vi "Sauna_9642_FPGA_Main.vi"() -> ()   [LabVIEW 2019]
uses:
  <vilib>/LabVIEW Targets/FPGA/cRIO/shared/nicrio_ModuleControls/nicrio_cRIO-9219_ConversionTime.ctl
  <vilib>/LabVIEW Targets/FPGA/cRIO/shared/nicrio_ModuleControls/nicrio_cRIO-9219_FullBridgeRange.ctl
  <vilib>/rvi/eio/common/nirviEmuTemplatePropertySet_noerrors.vi
  <vilib>/rvi/Emulation/niFpgaGetClockAttributes.vi
  <vilib>/rvi/Emulation/niFpgaSctlEmulationGetInTimedLoop.vi
  <vilib>/rvi/Emulation/niFpgaEmulationReportErrorSimple.vi
  <vilib>/rvi/Emulation/niFpgaProcessEmulError.vi
  <vilib>/rvi/eio/common/nirviEmuTemplateMethod_errors.vi
  <vilib>/rvi/Emulation/niFpgaCriticalErrorInLSC.vi
  <vilib>/eio/EIOPropertyNode/EIOPropertyNode.xnode
  <vilib>/eio/EIONode/EIONode.xnode
  <vilib>/eio/EIOMethodNode/EIOMethodNode.xnode
  <vilib>/rvi/eio/common/nirviEmuTemplatePropertyGet_errors.vi
  <vilib>/rvi/eio/common/nirviEmuTemplatePropertyGet_noerrors.vi
  <vilib>/rvi/eio/common/nirviEmuTemplatePropertySet_errors.vi
panel:
  in  "WaitForIRQ_\nAck":bool=TRUE
  in  "Kiuas LED":bool
  in  "Aromi LED":bool
  in  "Löyly LED":bool
  in  "Löyly Valve":bool
  in  "Aromi Pump":bool
  in  "Aromi Pump Enable":bool
  out "Kiuas Switch":bool
  in  "Löyly Valve Enable":bool
  out "Aromi Switch":bool
  out "Löyly Switch":bool
  in  "Pump Direction":bool
  in  "Pump Cycle":u32 caption="Count(uSec)"
  out "FPGA Error Out":errorcluster
  out "9219 Output":T1
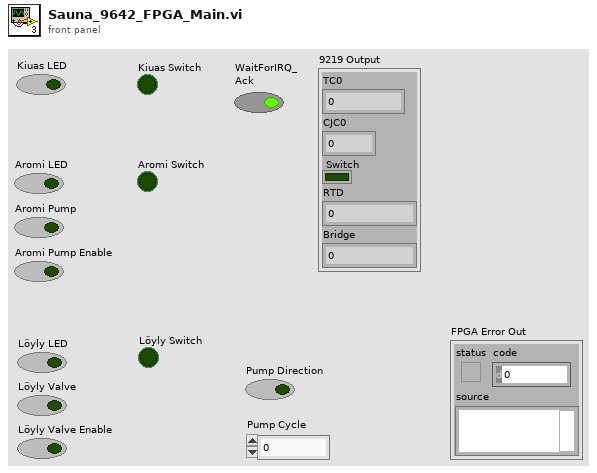
[diagram p1: front panel]
types:
  T1 = cluster{"TC0":fxp<+/-,32,-1>, "CJC0":fxp<+/-,32,-1>, "Switch":bool, "RTD":fxp<+,32,14>, "Bridge":fxp<+/-,32,-1>}
  T2 = typedef "nicrio_cRIO-9219_ConversionTime.ctl" = enum8{"High Speed", "Best 60 Hz Rejection", "Best 50 Hz Rejection", "High Resolution"}
  T3 = typedef "nicrio_cRIO-9219_FullBridgeRange.ctl" = u8
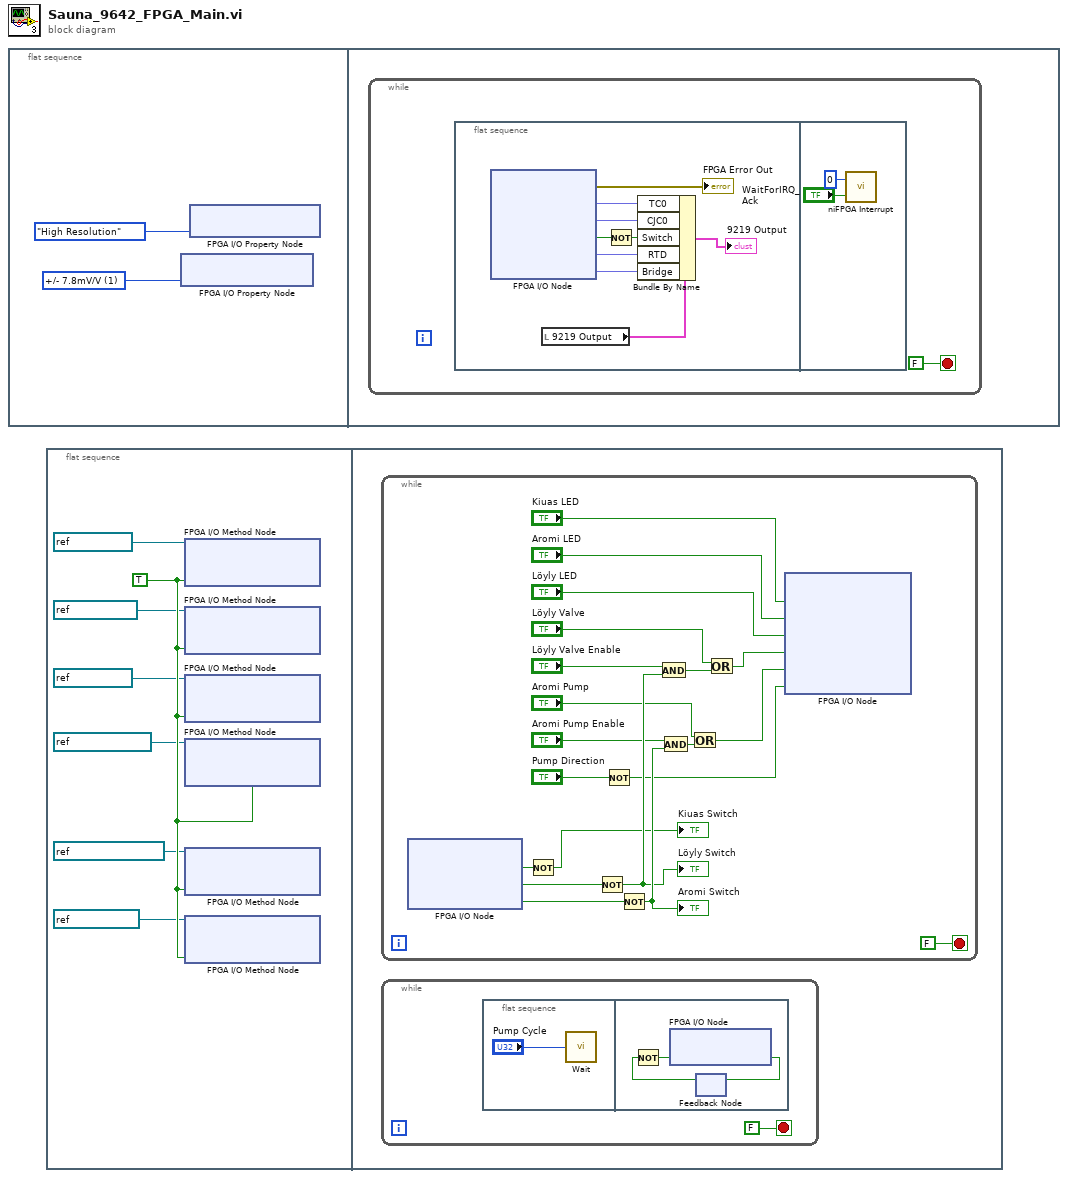
[diagram p0: block diagram]
diagram:
  n1 = flat-sequence {
    frame #0 {
      w2 = T3 1 items=["+/- 62.5mV/V", "+/- 7.8mV/V"] ("Full Bridge Range")
      n2 = xnode "FPGA I/O Property Node"("Full Bridge Range"=w2) -> ()  [unwired: 1 in, 1 out]
      n3 = xnode "FPGA I/O Property Node"("Conversion Time"=nicrio_cRIO-9219_ConversionTime."High Resolution") -> ()  [unwired: 1 in, 1 out]
    }
    frame #1 {
      n4 = while {
        stop <- FALSE stop-if-true
        n5 = flat-sequence {
          frame #0 {
            n6 = xnode "FPGA I/O Node"() -> ("error out"=→"FPGA Error Out":errorcluster, "Mod2/CH0"=w11:fxp<+/-,32,-1>, "Mod2/CJC0"=w10:fxp<+/-,32,-1>, "Mod2/CH1"=w5:bool, "Mod2/CH2"=w6:fxp<+,32,14>, "Mod2/CH3"=w7:fxp<+/-,32,-1>)  [unwired: 6 in, 5 out]
            n7 = local read "9219 Output"() -> (w8:T1)
            n8 = Not(x=w5) -> (.not. x?=w4:bool)
            n9 = Bundle By Name(cluster=w8, "TC0"=w11, "CJC0"=w10, "Switch"=w4, "RTD"=w6, "Bridge"=w7) -> (→"9219 Output":T1)
          }
          frame #1 {
            n10 = call <vilib>:"niFPGA Interrupt.vi"("Wait Until Cleared (F)"="WaitForIRQ_\nAck", "IRQ Number (0)"=u8 0 ("IRQ Bit (0-31)")) -> ()  [unwired: 1 in]
          }
        }
      }
    }
  }
  n11 = flat-sequence {
    frame #0 {
      w21 = TRUE ("Enable")
      n12 = xnode "FPGA I/O Method Node"("FPGA I/O In"=refnum<k21> "Kiuas LED" ("FPGA I/O"), "Enable"=w21) -> ()  [unwired: 1 out]
      n13 = xnode "FPGA I/O Method Node"("FPGA I/O In"=refnum<k21> "Aromi LED" ("FPGA I/O"), "Enable"=w21) -> ()  [unwired: 1 out]
      n14 = xnode "FPGA I/O Method Node"("FPGA I/O In"=refnum<k21> "Löyly LED" ("FPGA I/O"), "Enable"=w21) -> ()  [unwired: 1 out]
      n15 = xnode "FPGA I/O Method Node"("FPGA I/O In"=refnum<k21> "Pump Enable" ("FPGA I/O"), "Enable"=w21) -> ()  [unwired: 1 out]
      n16 = xnode "FPGA I/O Method Node"("FPGA I/O In"=refnum<k21> "Pump Direction" ("FPGA I/O"), "Enable"=w21) -> ()  [unwired: 1 out]
      n17 = xnode "FPGA I/O Method Node"("FPGA I/O In"=refnum<k21> "Pump Step" ("FPGA I/O"), "Enable"=w21) -> ()  [unwired: 1 out]
    }
    frame #1 {
      n18 = while {
        stop <- FALSE stop-if-true
        n19 = xnode "FPGA I/O Node"() -> ("Kiuas Switch"=w39:bool, "Löyly Switch"=w29:bool, "Aromi Switch"=w38:bool)  [unwired: 3 in, 3 out]
        n20 = Not(x=w39) -> (.not. x?=→"Kiuas Switch":bool)
        n21 = Not(x=w29) -> (.not. x?=w33:bool)
        "Löyly Switch" <- w33
        n22 = Not(x="Pump Direction") -> (.not. x?=w22:bool)
        n23 = Not(x=w38) -> (.not. x?=w36:bool)
        "Aromi Switch" <- w36
        n24 = And(x="Löyly Valve Enable", y=w33) -> (x .and. y?=w34:bool)
        n25 = And(x="Aromi Pump Enable", y=w36) -> (x .and. y?=w35:bool)
        n26 = Or(x="Aromi Pump", y=w35) -> (x .or. y?=w31:bool)
        n27 = Or(x="Löyly Valve", y=w34) -> (x .or. y?=w26:bool)
        n28 = xnode "FPGA I/O Node"("Kiuas LED"="Kiuas LED", "Aromi LED"="Aromi LED", "Löyly LED"="Löyly LED", "Löyly Valve"=w26, "Pump Enable"=w31, "Pump Direction"=w22) -> ()  [unwired: 6 in, 6 out]
      }
      n29 = while {
        stop <- FALSE stop-if-true
        n30 = flat-sequence {
          frame #0 {
            n31 = call "Wait"("Count(Ticks)"="Pump Cycle") -> ()  [unwired: 1 out]
          }
          frame #1 {
            n32 = feedback #1() -> (w45:bool)  [unwired: 1 in]
            n33 = Not(x=w45) -> (.not. x?=w44:bool)
            n34 = xnode "FPGA I/O Node"("Pump Step"=w44) -> ()  [unwired: 1 in, 1 out]
            n35 = feedback-in #1(w44) -> ()
          }
        }
      }
    }
  }
